vi "INSERT_CALIBRATION.vi"(8 "error in (no error)":errorcluster, 11 "C&C Data in":T1={"Hardware Configuration"={"COM Port"="", "Reference Distance"=0.0, "Sensor SN"=""}, "Logging Configuration"={"Log File Base Path"=path "", "Datafile Ref"=refnum, "Database Ref"=refnum}, "UI Refs"={"Start Ref"=refnum, "Settings Ref"=refnum, "Stop Ref"=refnum, "Exit Ref"=refnum, "Status Ref"=refnum, "Data Ref"=refnum, "StatusBox Ref"=refnum, "Location Ref"=refnum, "Operator Ref"=refnum, "Time Ref"=refnum, "Test in Progess Ref"=refnum}, "Calibration Data"={"calibrationID"=0, "operatorID"=0, "sensorID"=0, "start_time"="", "end_time"="", "offset"=0.0, "offset_units"="", "ring_time"=0.0, "error"=0.0, "Passed"=0, "data_storage_location"="", "comments"=""}, "Time Elapsed"=0, "Samples Required"=480} {"Hardware Configuration"."Reference Distance" format="%.3g"}) -> (0 "error out":errorcluster, 2 "connection reference out":T4)   [LabVIEW 2018, in "MySQLTools.lvlib"]
doc: "Calibration data is input to the database as a cluster in the following format:\n\noperatorID(int)\nsensorID(int)\nstart_time(datetime) YYYY-MM-DD 00:00:00\nend_time(datetime) YYYY-MM-DD 00:00:00\noffset(float)\noffset_units(varchar(5))\nring_time(double)\nerror(float)\npassed(tinyint(4))\ndata_storage_location(varchar(200))\ncomments(varchar(500))"
uses:
  MySQLTools.lvlib
  <vilib>/addons/database/Connection.llb/Conn ObjectReference.ctl
  uWaveOffset/Settings/Settings.ctl
  uWaveOffset/Acquisition/Hardware Configuration.ctl
  uWaveOffset/Logging/Logging Configuration.ctl
  uWaveOffset/Controls/Location Ring.ctl
  uWaveOffset/Controls/Time Remaining.ctl
  <vilib>/addons/database/NI_Database_API.lvlib
  uWaveOffset/Acquisition/Acquisition.lvlib
  uWaveOffset/Logging/Logging.lvlib
  uWaveOffset/Settings/Settings.lvlib
panel:
  # "SELECT * FROM ostepdb.calibrations;\nINSERT INTO `ostepdb`.`calibrations` (`operatorID`, `sensorID`, `start_time`, `end_time`, `offset`, `offset_units`, `error`, `data_storage_location`,`passed`) VALUES ('2', '1', '2015-12-20 10:01:00', '2015-12-20 10:01:00', '.0011', 'm', '0.001', 'C:\\\\Data\\\\TestLocation','1');"
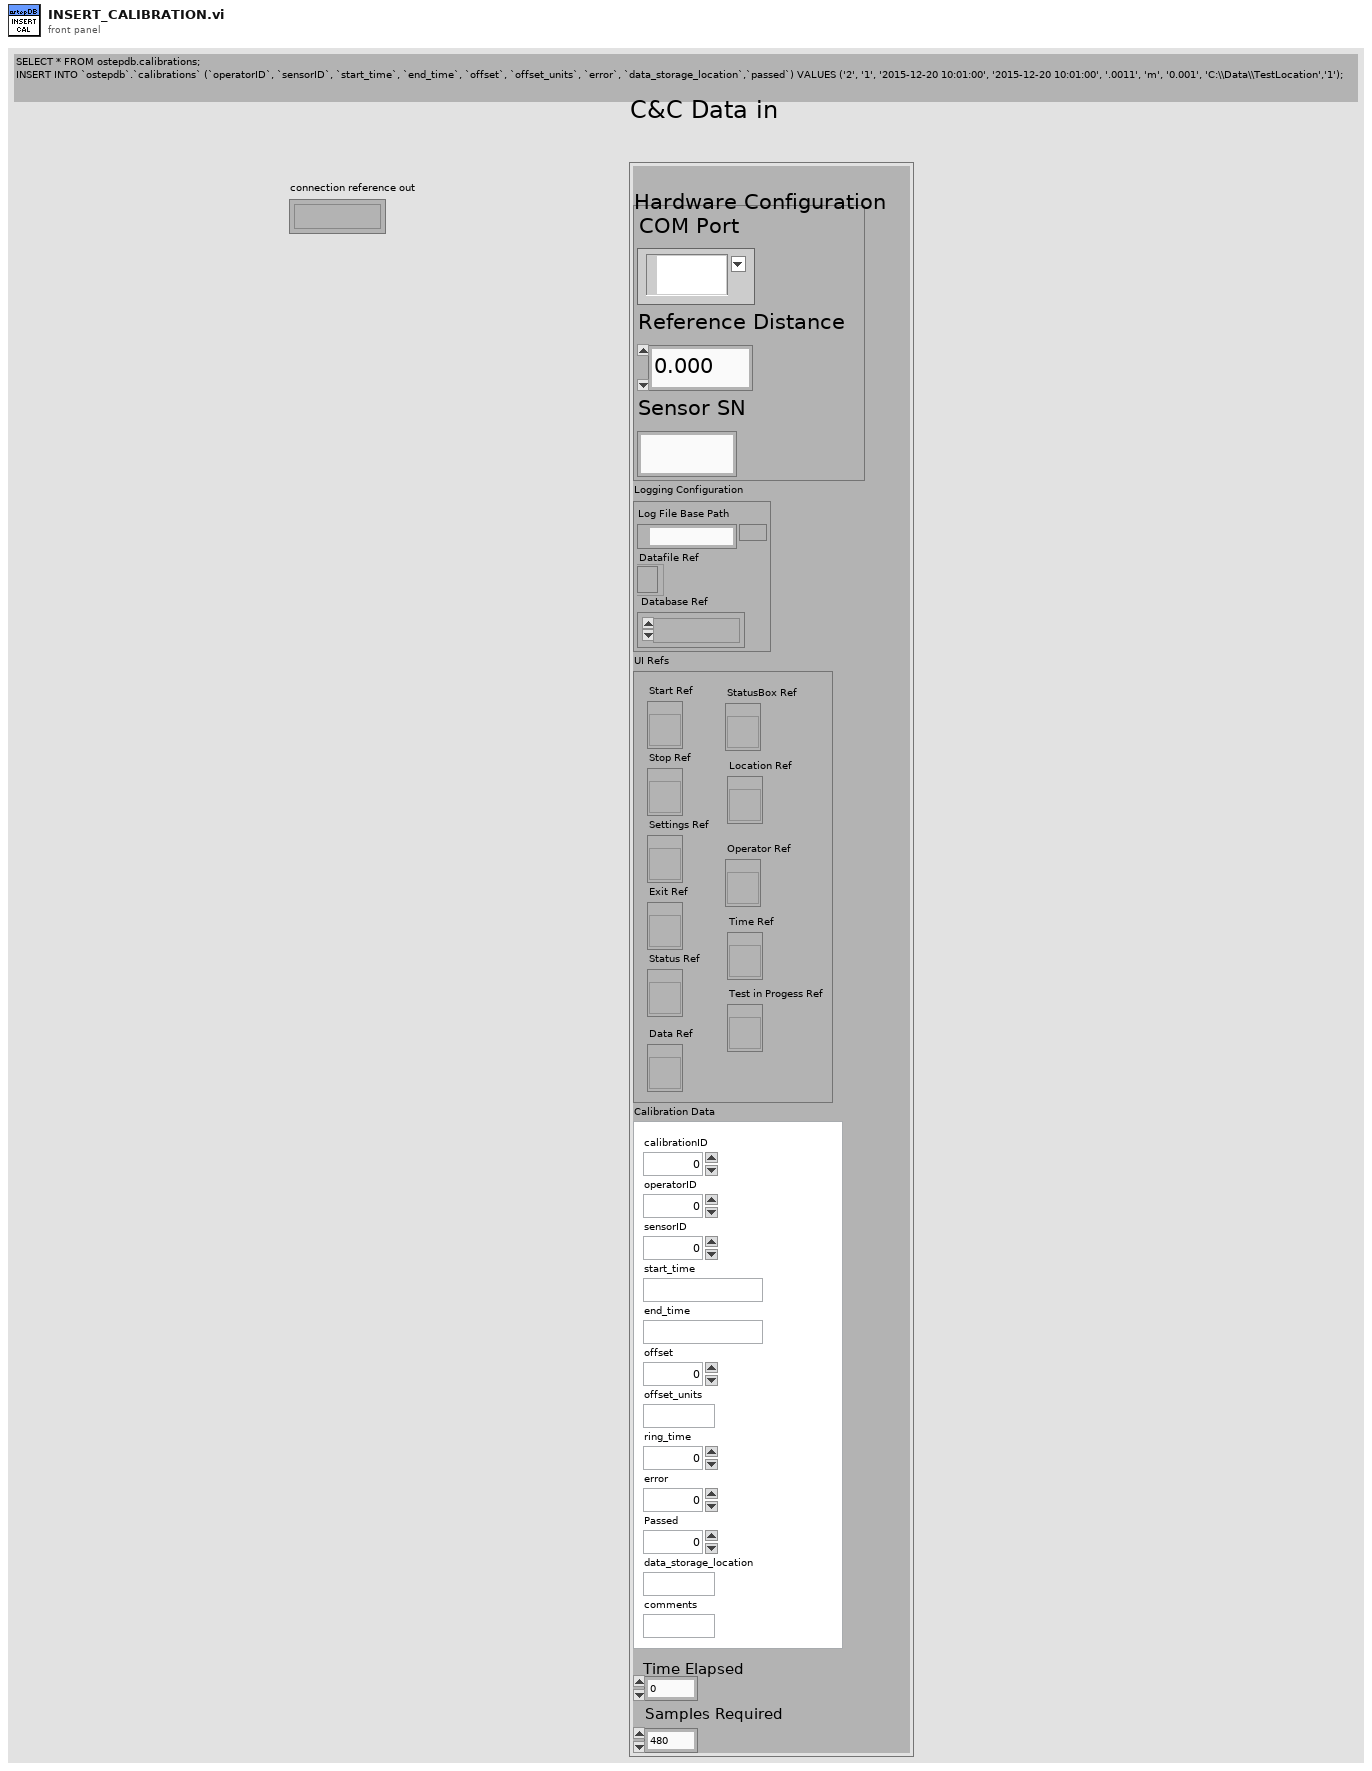
[diagram p1: front panel]
types:
  T1 = typedef "Settings.lvlib/Settings.ctl" = cluster{"Hardware Configuration":T2, "Logging Configuration":T3, "UI Refs":cluster{"Start Ref":refnum<vi>, "Settings Ref":refnum<vi>, "Stop Ref":refnum<vi>, "Exit Ref":refnum<vi>, "Status Ref":refnum<vi>, "Data Ref":refnum<vi>, "StatusBox Ref":refnum<vi>, "Location Ref":refnum<vi>, "Operator Ref":refnum<vi>, "Time Ref":refnum<vi>, "Test in Progess Ref":refnum<vi>}, "Calibration Data":cluster{"calibrationID":u16, "operatorID":u16, "sensorID":u16, "start_time":string, "end_time":string, "offset":dbl, "offset_units":string, "ring_time":dbl, "error":dbl, "Passed":u8, "data_storage_location":string, "comments":string}, "Time Elapsed":u16, "Samples Required":u16}
  T2 = typedef "Acquisition.lvlib/Hardware Configuration.ctl" = cluster{"COM Port":refnum<visa-resource-name>, "Reference Distance":dbl, "Sensor SN":string}
  T3 = typedef "Logging.lvlib/Logging Configuration.ctl" = cluster{"Log File Base Path":path, "Datafile Ref":refnum<file>, "Database Ref":T4}
  T4 = typedef "NI_Database_API.lvlib/Conn ObjectReference.ctl" = refnum<k1>
  T5 = cluster{"calibrationID":u16, "operatorID":u16, "sensorID":u16, "start_time":string, "end_time":string, "offset":dbl, "offset_units":string, "ring_time":dbl, "error":dbl, "Passed":u8, "data_storage_location":string, "comments":string}
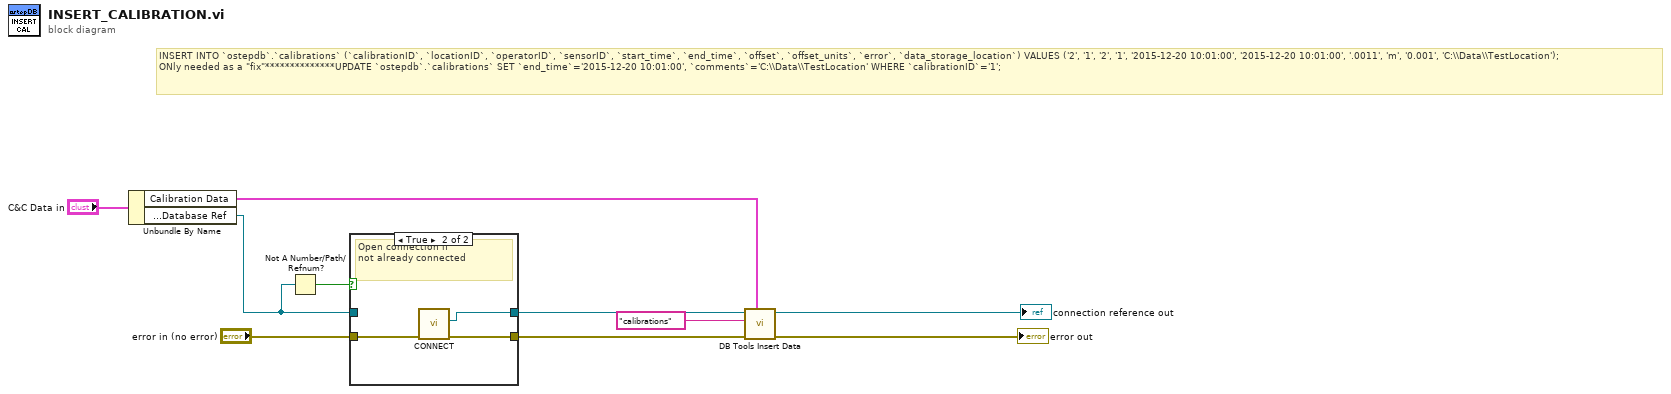
[diagram p0: block diagram]
diagram:
  # "INSERT INTO `ostepdb`.`calibrations` (`calibrationID`, `locationID`, `operatorID`, `sensorID`, `start_time`, `end_time`, `offset`, `offset_units`, `error`, `data_storage_location`) VALUES ('2', '1', '2', '1', '2015-12-20 10:01:00', '2015-12-20 10:01:00', '.0011', 'm', '0.001', 'C:\\\\Data\\\\TestLocation');\nONly needed as a \"fix\"**************UPDATE `ostepdb`.`calibrations` SET `end_time`='2015-12-20 10:01:00', `comments`='C:\\\\Data\\\\TestLocation' WHERE `calibrationID`='1';"
  n1 = Unbundle By Name("C&C Data in") -> ("Calibration Data"=w3:T5, "Logging Configuration.Database Ref"=w1:T4)
  n2 = Not A Number/Path/Refnum?(number/path/refnum=w1) -> (NaN/Path/Refnum?=w5:bool)
  n3 = case shown="True" w5 {
    tunnel: "error in (no error)" -> [w11 w15]
    tunnel: [w11 w14] -> w8
    tunnel: [w12 w13] -> w7
    tunnel: w1 -> [w12 _]
    frame False {
      # "If already connected,\npassthru reference"
    }
    frame True {
      # "Open connection if\nnot already connected"
      n4 = call "CONNECT.vi"("error in (no error)"=w15) -> ("error out"=w14:errorcluster, "connection ref out"=w13:T4)  [unwired: 9 in]
    }
  }
  n5 = call <vilib>:"DB Tools Insert Data.vi"("data"=w3, "error in (no error)"=w8, "table"="calibrations", "connection reference"=w7) -> ("error out"=→"error out":errorcluster, "connection reference out"=→"connection reference out":T4)  [unwired: 6 in]
